vi "FABR-Init Frequency.vi"(0 "Stimulus":T1={"Ear"=enum."Left", "Start (kHz)"=20.0, "Stop (kHz)"=80.0, "Step (oct)"=5.0, "Start (dB)"=20, "Stop (dB)"=80, "Step (dB)"=5, "Rep rate (/sec)"=30.0, "Alternate Polarity"=FALSE, "Skip (oct)"=0.0} {"Start (kHz)" step=5.0; "Start (dB)" step=5}, 5 "Runtime in":T2, 11 "error in (no error)":errorcluster) -> (4 "Stimulus thru":T1={"Ear"=enum."Left", "Start (kHz)"=20.0, "Stop (kHz)"=80.0, "Step (oct)"=5.0, "Start (dB)"=20, "Stop (dB)"=80, "Step (dB)"=5, "Rep rate (/sec)"=30.0, "Alternate Polarity"=FALSE, "Skip (oct)"=0.0} {"Start (kHz)" step=5.0; "Start (dB)" step=5}, 6 "Runtime out":T2, 8 "SCL":T3[](array[typedef]), 15 "error out":errorcluster)   [LabVIEW 2020]
uses:
  Typedefs/FABR-Stimulus.ctl
  Typedefs/FABR-Stimulus Condition.ctl
  Typedefs/FABR-Runtime Data.ctl
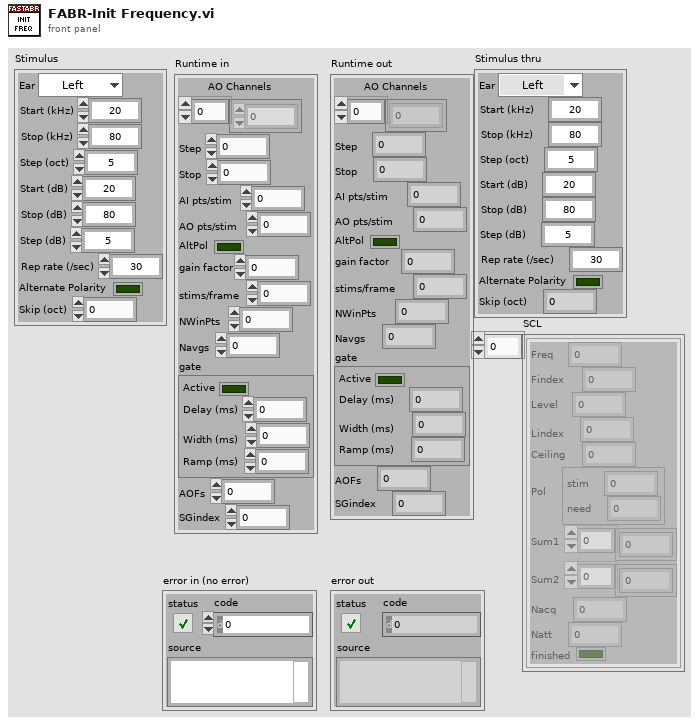
[diagram p1: front panel]
types:
  T1 = typedef "FABR-Stimulus.ctl" = cluster{"Ear":enum16{"Right", "Left"}, "Start (kHz)":dbl, "Stop (kHz)":dbl, "Step (oct)":dbl, "Start (dB)":i32, "Stop (dB)":i32, "Step (dB)":i32, "Rep rate (/sec)":dbl, "Alternate Polarity":bool, "Skip (oct)":dbl}
  T2 = typedef "FABR-Runtime Data.ctl" = cluster{"AO Channels":i32[], "Step":dbl, "Stop":i32, "AI pts/stim":i32, "AO pts/stim":i32, "AltPol":bool, "gain factor":dbl, "stims/frame":i32, "NWinPts":i32, "Navgs":i32, "gate":cluster{"Active":bool, "Delay (ms)":dbl, "Width (ms)":dbl, "Ramp (ms)":dbl}, "AOFs":dbl, "SGindex":i32}
  T3 = typedef "FABR-Stimulus Condition.ctl" = cluster{"Freq":dbl, "Findex":i32, "Level":dbl, "Lindex":i32, "Ceiling":dbl, "Pol":cluster{"stim":i32, "need":i32}, "Sum1":dbl[], "Sum2":dbl[], "Nacq":i32, "Natt":i32, "finished":bool}
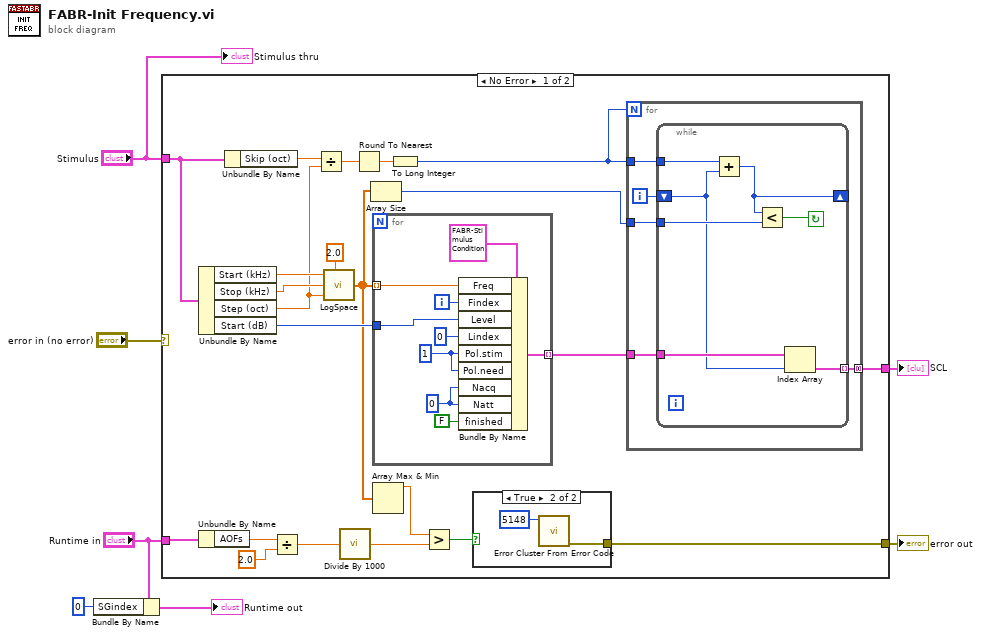
[diagram p0: block diagram]
diagram:
  n1 = Bundle By Name(cluster="Runtime in", "SGindex"=0) -> (→"Runtime out":T2)
  n2 = case shown="No Error" "error in (no error)" {
    selector: "error in (no error)" -> [_ w53]
    tunnel: "Stimulus" -> [w17 _]
    tunnel: [w18 _] -> w4
    tunnel: [w9 w53] -> w2
    tunnel: "Runtime in" -> [w16 _]
    frame No Error {
      n3 = Unbundle By Name(w17) -> ("Start (kHz)"=w28:dbl, "Stop (kHz)"=w27:dbl, "Step (oct)"=w25:dbl, "Start (dB)"=w26:i32)
      n4 = Unbundle By Name(w16) -> ("AOFs"=w15:dbl)
      n5 = Unbundle By Name(w17) -> ("Skip (oct)"=w24:dbl)
      n6 = Divide(x=w15, y=2.0) -> (x/y=w13:dbl)
      n7 = Divide(x=w24, y=w25) -> (x/y=w23:dbl)
      n8 = call "LogSpace.vi"("Start"=w28, "Base"=2.0, "Stop"=w27, "Step"=w25) -> ("Array"=w12:dbl[])  [unwired: 2 in, 1 out]
      n9 = call "Divide By 1000.vi"("X"=w13) -> ("X/1000"=w8:dbl)
      n10 = Round To Nearest(number=w23) -> (nearest integer value=w22:dbl)
      n11 = Array Size(array=w12) -> (size(s)=w20:i32)
      n12 = for {
        tunnel: w12 -> [w51] mode=indexing
        tunnel: w26 -> [w49]
        tunnel: [w45] -> w19 mode=indexing
        i -> [w50]
        w47 = 0 ("Nacq")
        w44 = 1 ("Pol")
        n13 = Bundle By Name(cluster=T3 {"Freq"=0.0, "Findex"=0, "Level"=0.0, "Lindex"=0, "Ceiling"=0.0, "Pol"={"stim"=0, "need"=0}, "Sum1"=[], "Sum2"=[], "Nacq"=0, "Natt"=0, "finished"=FALSE} ("SC"), "Freq"=w51, "Findex"=w50, "Level"=w49, "Lindex"=0, "Pol.stim"=w44, "Pol.need"=w44, "Nacq"=w47, "Natt"=w47, "finished"=FALSE) -> (w45:T3)
      }
      n14 = Array Max & Min(array=w12) -> (max value=w11:dbl)  [unwired: 3 out]
      n15 = To Long Integer(number=w22) -> (32bit integer=w21:i32)
      n16 = Greater?(x=w11, y=w8) -> (0:w10:bool)
      n17 = case shown="True" w10 {
        tunnel: [_ w31] -> w9
        frame False {
        }
        frame True {
          n18 = call <vilib>:"Error Cluster From Error Code.vi"("error code (0)"=5148) -> ("error out"=w31:errorcluster)  [unwired: 8 in]
        }
      }
      n19 = for {
        N: w21 -> [_]
        tunnel: w21 -> [w36]
        tunnel: w20 -> [w34]
        tunnel: w19 -> [w33]
        tunnel: [w32] -> w18 mode=concatenating
        i -> [w35]
        n20 = while {
          tunnel: w36 -> [w43]
          shift-right: [w42] -> _
          shift-left: w35 -> [w38]
          tunnel: w34 -> [w41]
          tunnel: w33 -> [w39]
          tunnel: [w37] -> w32 mode=indexing
          stop <- w40 continue-if-true
          n21 = Add(x=w43, y=w38) -> (x+y=w42:i32)
          n22 = Less?(x=w42, y=w41) -> (x < y?=w40:bool)
          n23 = Index Array(array=w39, index=w38) -> (element=w37:T3)
        }
      }
    }
    frame Error {
    }
  }
  "SCL" <- w4
  "error out" <- w2
  "Stimulus thru" <- "Stimulus"
